vi "NextMonth.vi"(8 "error in (no error)":errorcluster, 11 "Calendar in":refnum<class "Calendar.lvclass">) -> (0 "error out":errorcluster, 3 "Calendar (dup)":refnum<class "Calendar.lvclass">)   [LabVIEW 2020, in "Calendar.lvclass"]
uses:
  Calendar.lvclass
  Calendar.lvclass/Calendar.ctl
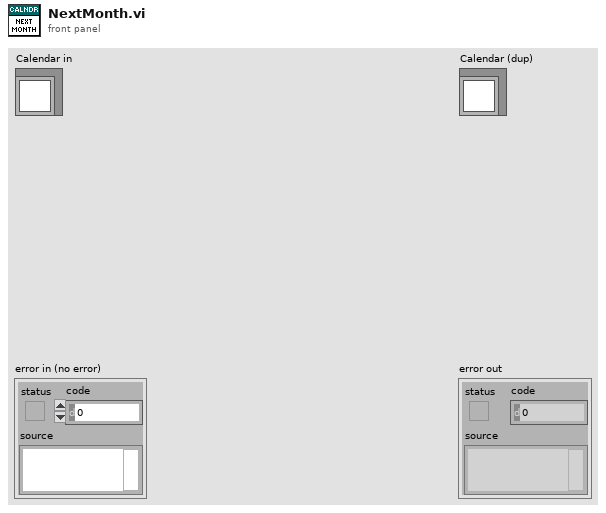
[diagram p1: front panel]
types:
  T1 = typedef "Calendar.lvclass/State Data.ctl" = cluster{"Current Date":timestamp, "First Day of Week":T2, "Color":cluster{"Selector Background":u32, "Selector Text":u32, "Days of Week Background":u32, "Days of Week Text":u32, "Calendar Background":u32, "Calendar Text":u32, "Calendar Selection Background":u32, "Calendar Selection Text":u32}, "Visible":cluster{"Today Selector Visible":bool, "Month-Year Selector Visible":bool}}
  T2 = typedef "Calendar.lvclass/DaysOfWeek.ctl" = enum16{"Sunday", "Monday", "Tuesday", "Wednesday", "Thursday", "Friday", "Saturday"}
  T3 = typedef "LVDateTimeRec.ctl" = cluster{"fractional second":dbl, "second":i32, "minute":i32, "hour":i32, "day of month":i32, "month":i32, "year":i32, "day of week":i32, "day of year":i32, "DST":i32}
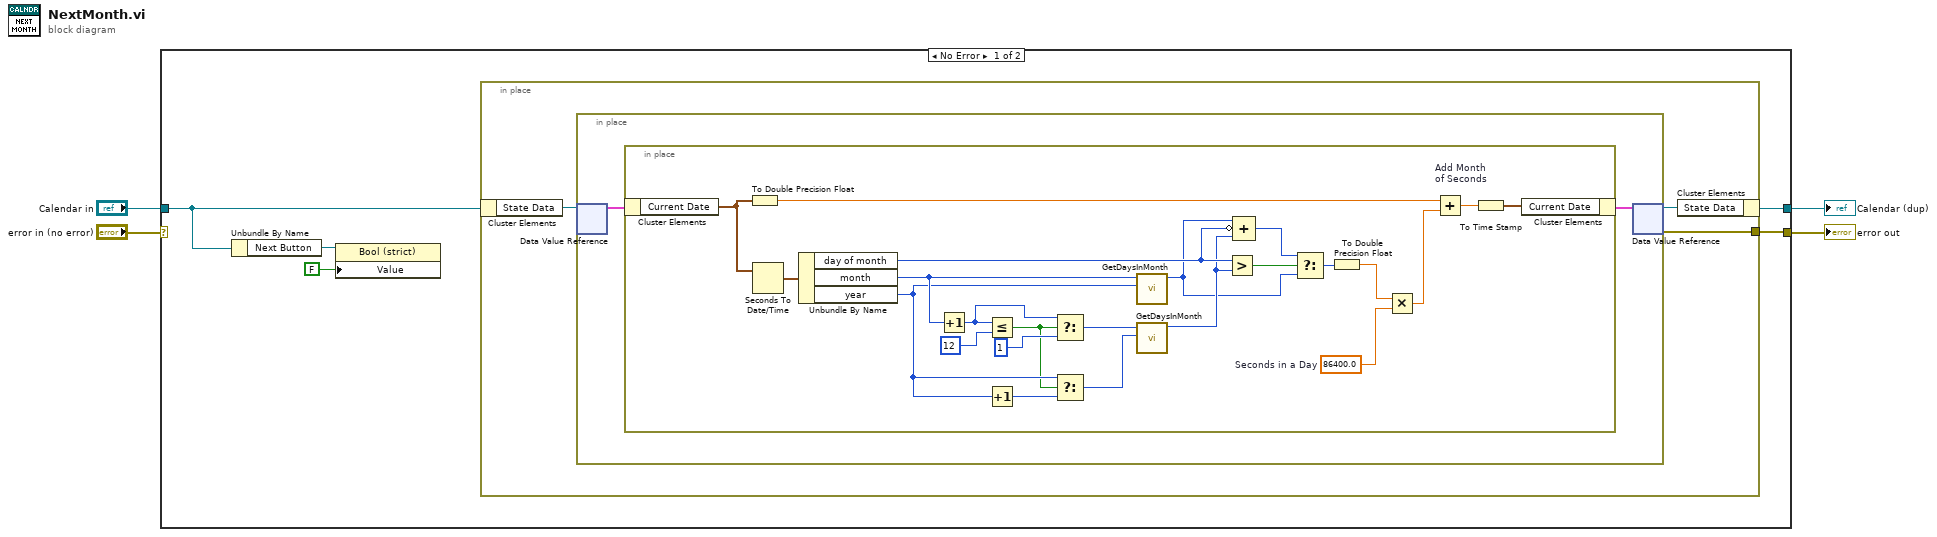
[diagram p0: block diagram]
diagram:
  n1 = case shown="No Error" "error in (no error)" {
    selector: "error in (no error)" -> [_ w39]
    tunnel: [w8 w39] -> w3
    tunnel: [w9 w38] -> w1
    tunnel: "Calendar in" -> [w5 w38]
    frame No Error {
      n2 = Unbundle By Name(w5) -> ("Next Button"=w7:refnum<vi>)
      n3 = property class="Bool (strict)"(reference=w7, "Value"=FALSE) -> ()  [unwired: 1 in, 2 out]
      n4 = in-place {
        in-place-border: [w10] -> w8
        n5 = in-place-cluster #1(w5) -> ("State Data"=w12:refnum<data-value>)
        n6 = in-place {
          n7 = in-place-dvr #2(w12) -> (w14:T1)  [unwired: 1 out]
          n8 = in-place {
            w35 = 86400.0  # Seconds in a Day
            n9 = in-place-cluster #3(w14) -> ("Current Date"=w37:timestamp)
            n10 = To Double Precision Float(number=w37) -> (double precision float=w33:dbl)
            n11 = Seconds To Date/Time(time stamp (now)=w37) -> (date time rec=w36:T3)  [unwired: 1 in]
            n12 = Unbundle By Name(w36) -> ("day of month"=w21:i32, "month"=w30:i32, "year"=w26:i32)
            n13 = Increment(x=w30) -> (x+1=w28:i32)
            n14 = Less Or Equal?(x=w28, y=12 ("upper limit")) -> (x <= y?=w25:bool)
            n15 = Increment(x=w26) -> (x+1=w24:i32)
            n16 = Select(t=w28, s=w25, f=1) -> (s? t:f=w23:i32)
            n17 = Select(t=w26, s=w25, f=w24) -> (s? t:f=w22:i32)
            n18 = call "GetDaysInMonth.vi"("Year"=w26, "Month"=w30) -> ("Number of Days in Month"=w17:i32)  [unwired: 8 in, 1 out]
            n19 = call "GetDaysInMonth.vi"("Year"=w22, "Month"=w23) -> ("Number of Days in Month"=w19:i32)  [unwired: 8 in, 1 out]
            n20 = Greater?(x=w21, y=w19) -> (0:w20:bool)
            n21 = Compound Arithmetic op=ADD(w17, invert w21, w19) -> (w18:i32)
            n22 = Select(t=w18, s=w20, f=w17) -> (s? t:f=w16:i32)
            n23 = To Double Precision Float(number=w16) -> (double precision float=w15:dbl)
            n24 = Multiply(x=w15, y=w35) -> (x*y=w32:dbl)
            n25 = Add "Add Month\nof Seconds"(x=w33, y=w32) -> (x+y=w31:dbl)
            n26 = To Time Stamp(1:w31) -> (0:w34:timestamp)
            n27 = in-place-cluster #3("Current Date"=w34) -> (w13:T1)
          }
          n28 = in-place-dvr #2(w13) -> (w11:refnum<data-value>, w10:errorcluster)
        }
        n29 = in-place-cluster #1("State Data"=w11) -> (w9:refnum<class "Calendar.lvclass">)
      }
    }
    frame Error {
    }
  }
  "error out" <- w3
  "Calendar (dup)" <- w1
